vi "Robot Main.vi"() -> ()   [LabVIEW 2018]
doc: "Robot Main serves as the primary scheduler for your command and control robotics program. It should not be necessary to modify this VI. Instead, you should add your code to the VIs called from Robot Main - Teleop, Autonomous, and SubSystems."
uses:
  <vilib>/Rock Robotics/WPI/Camera/WPI_CameraImageSize.ctl
  Drive/Implementation/Drive Operations.ctl
  <vilib>/Rock Robotics/SystemInterfaces/NetworkCommunication/NetComm_UsageReport_ResourceType.ctl
  Framework/Robot Global Data.vi
  LattePanda/Implementation/LattePanda Published Globals.vi
  <vilib>/Rock Robotics/Network Tables/NT Write Number.vi
  <vilib>/Rock Robotics/Network Tables/NT Read String.vi
  <vilib>/Rock Robotics/Network Tables/NT Write Variant.vi
panel:
  out "Path Data":refnum<vi>[](array[refnum])
  out "LattePanda Connected":bool
  in  "Operation":T1=enum."Immediate"
  in  "Image Size":T2=enum."320x240"
  in  "Finish":bool
  # "1. Get the camera mounted on the back\n2. Clean up Elevator Teleop"
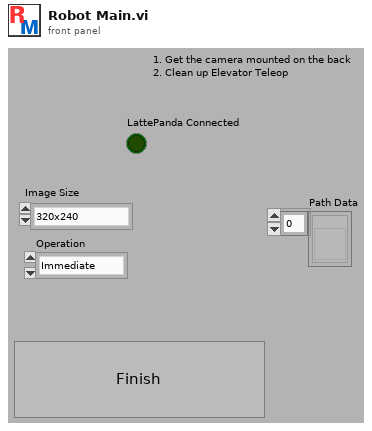
[diagram p1: front panel]
types:
  T1 = typedef "Drive Operations.ctl" = enum16{"Reserve", "Read Current", "Immediate", "J-Turn", "Play Back From Log", "Auto-Align"}
  T2 = typedef "WPI_CameraImageSize.ctl" = enum16{"640x480", "320x240", "160x120", "Custom"}
  T3 = typedef "NetComm_UsageReport_ResourceType.ctl" = enum8{"Controller", "Module", "Language", "CANPlugin", "Accelerometer", "ADXL345", "AnalogChannel", "AnalogTrigger", "AnalogTriggerOutput", "CANJaguar", "Compressor", "Counter", "Dashboard", "DigitalInput", "DigitalOutput", "DriverStationCIO", "DriverStationEIO", "DriverStationLCD", "Encoder", "GearTooth", "Gyro", "I2C", "Framework", "Jaguar", "Joystick", "Kinect", "KinectStick", "PIDController", "Preferences", "PWM", "Relay", "RobotDrive", "SerialPort", "Servo", "Solenoid", "SPI", "Task", "Ultrasonic", "Victor", "Button", "Command", "AxisCamera", "PCVideoServer", "SmartDashboard", "Talon", "HiTechnicColorSensor", "HiTechnicAccel", "HiTechnicCompass", "SRF08", "AnalogOutput", "Victor SP", "Talon SRX", "CAN Talon SRX", "ADXL362 Accel", "ADXRS450 Gyro", "Rev SPARK", "Mindsensors SD540", "Digital Filter", "ADIS16448", "PDP", "PCM", "PigeonIMU", "Nidec Brushless", "CTRE CANifier", "CTRE Future 0", "CTRE Future 1", "CTRE Future 2", "CTRE Future 3", "CTRE Future 4", "CTRE Future 5", "CTRE Future 6", "Linear Filter", "Xbox Controller", "USB Camera", "NavX", "Pixy", "Pixy2", "ScanseSweep", "Shuffleboard", "CAN", "Digilent DMC60", "PWM Victor SPX", "Rev SPARK MAX PWM", "Rev SPARK MAX CAN", "ADIS16470"}
  T4 = cluster{"Segment Name":string, "Type":enum16{"Accel Straight", "Const Straight", "Blend", "Circle"}, "Traj Pos Points":cluster{"x":dbl, "y":dbl, "th":dbl}[], "Traj Vel Points":cluster{"V":dbl, "th":dbl}[], "Accel Index":i32, "Decel Index":i32}[]
  T5 = cluster{"Points":cluster{"x":dbl, "y":dbl, "th":dbl}[], "Trajectory Data":cluster{"Segment Name":string, "Type":enum16{"Accel Straight", "Const Straight", "Blend", "Circle"}, "Traj Pos Points":cluster{"x":dbl, "y":dbl, "th":dbl}[], "Traj Vel Points":cluster{"V":dbl, "th":dbl}[], "Accel Index":i32, "Decel Index":i32}[]}
  T6 = typedef "ADIS16448_IMU.lvlib/ADI_IMU_ADIS16448_IMUDevRef.ctl" = cluster{"DevStatus":errorcluster, "Handle":i32, "SPI Bus":T7, "Device Found":bool, "Device Ready":bool, "Yaw Axis":enum16{"X", "Y", "Z"}, "AHRS Algorithm":enum16{"Complementary", "Madgwick"}, "Serial":u16, "Lot ID 2":u16, "Lot ID 1":u16, "Bytes Per Sample":u16, "Calibrate On Open?":bool}
  T7 = typedef "spi_bus.ctl" = enum16{"SPI On-Board, CS0", "SPI On-Board, CS1", "SPI On-Board, CS2", "SPI On-Board, CS3", "SPI MXP", "Invalid"}
  T8 = typedef "WPI_JoystickDevRef.ctl" = cluster{"Device":T9}
  T9 = typedef "WPI_JoystickDeviceEnum.ctl" = enum16{"USB 0", "USB 1", "USB 2", "USB 3", "USB 4", "USB 5"}
  T10 = typedef "WPI_DriverStationMatch Info.ctl" = cluster{"Autonomous Elapsed Seconds":dbl, "TeleOp Elapsed Seconds":dbl, "Disabled Elapsed Seconds":dbl, "Visited Autonomous":bool, "Visited TeleOp":bool, "Visited Disabled":bool, "Autonomous Settings":cluster{"Autonomous Style":enum16{"Iterative", "Independent"}, "VI Refnum":refnum<vi>}}
  T11 = typedef "WPI_DriverStationDerivedRobotMode.ctl" = enum16{"Init", "Execute", "Stop"}
  T12 = typedef "WPI_DriverStationRobotMode2.ctl" = enum16{"Autonomous Disabled", "Autonomous Enabled", "Teleop Disabled", "Teleop Enabled", "Disconnected", "Finish", "Test Disabled", "Test Enabled", "Emergency Stopped"}
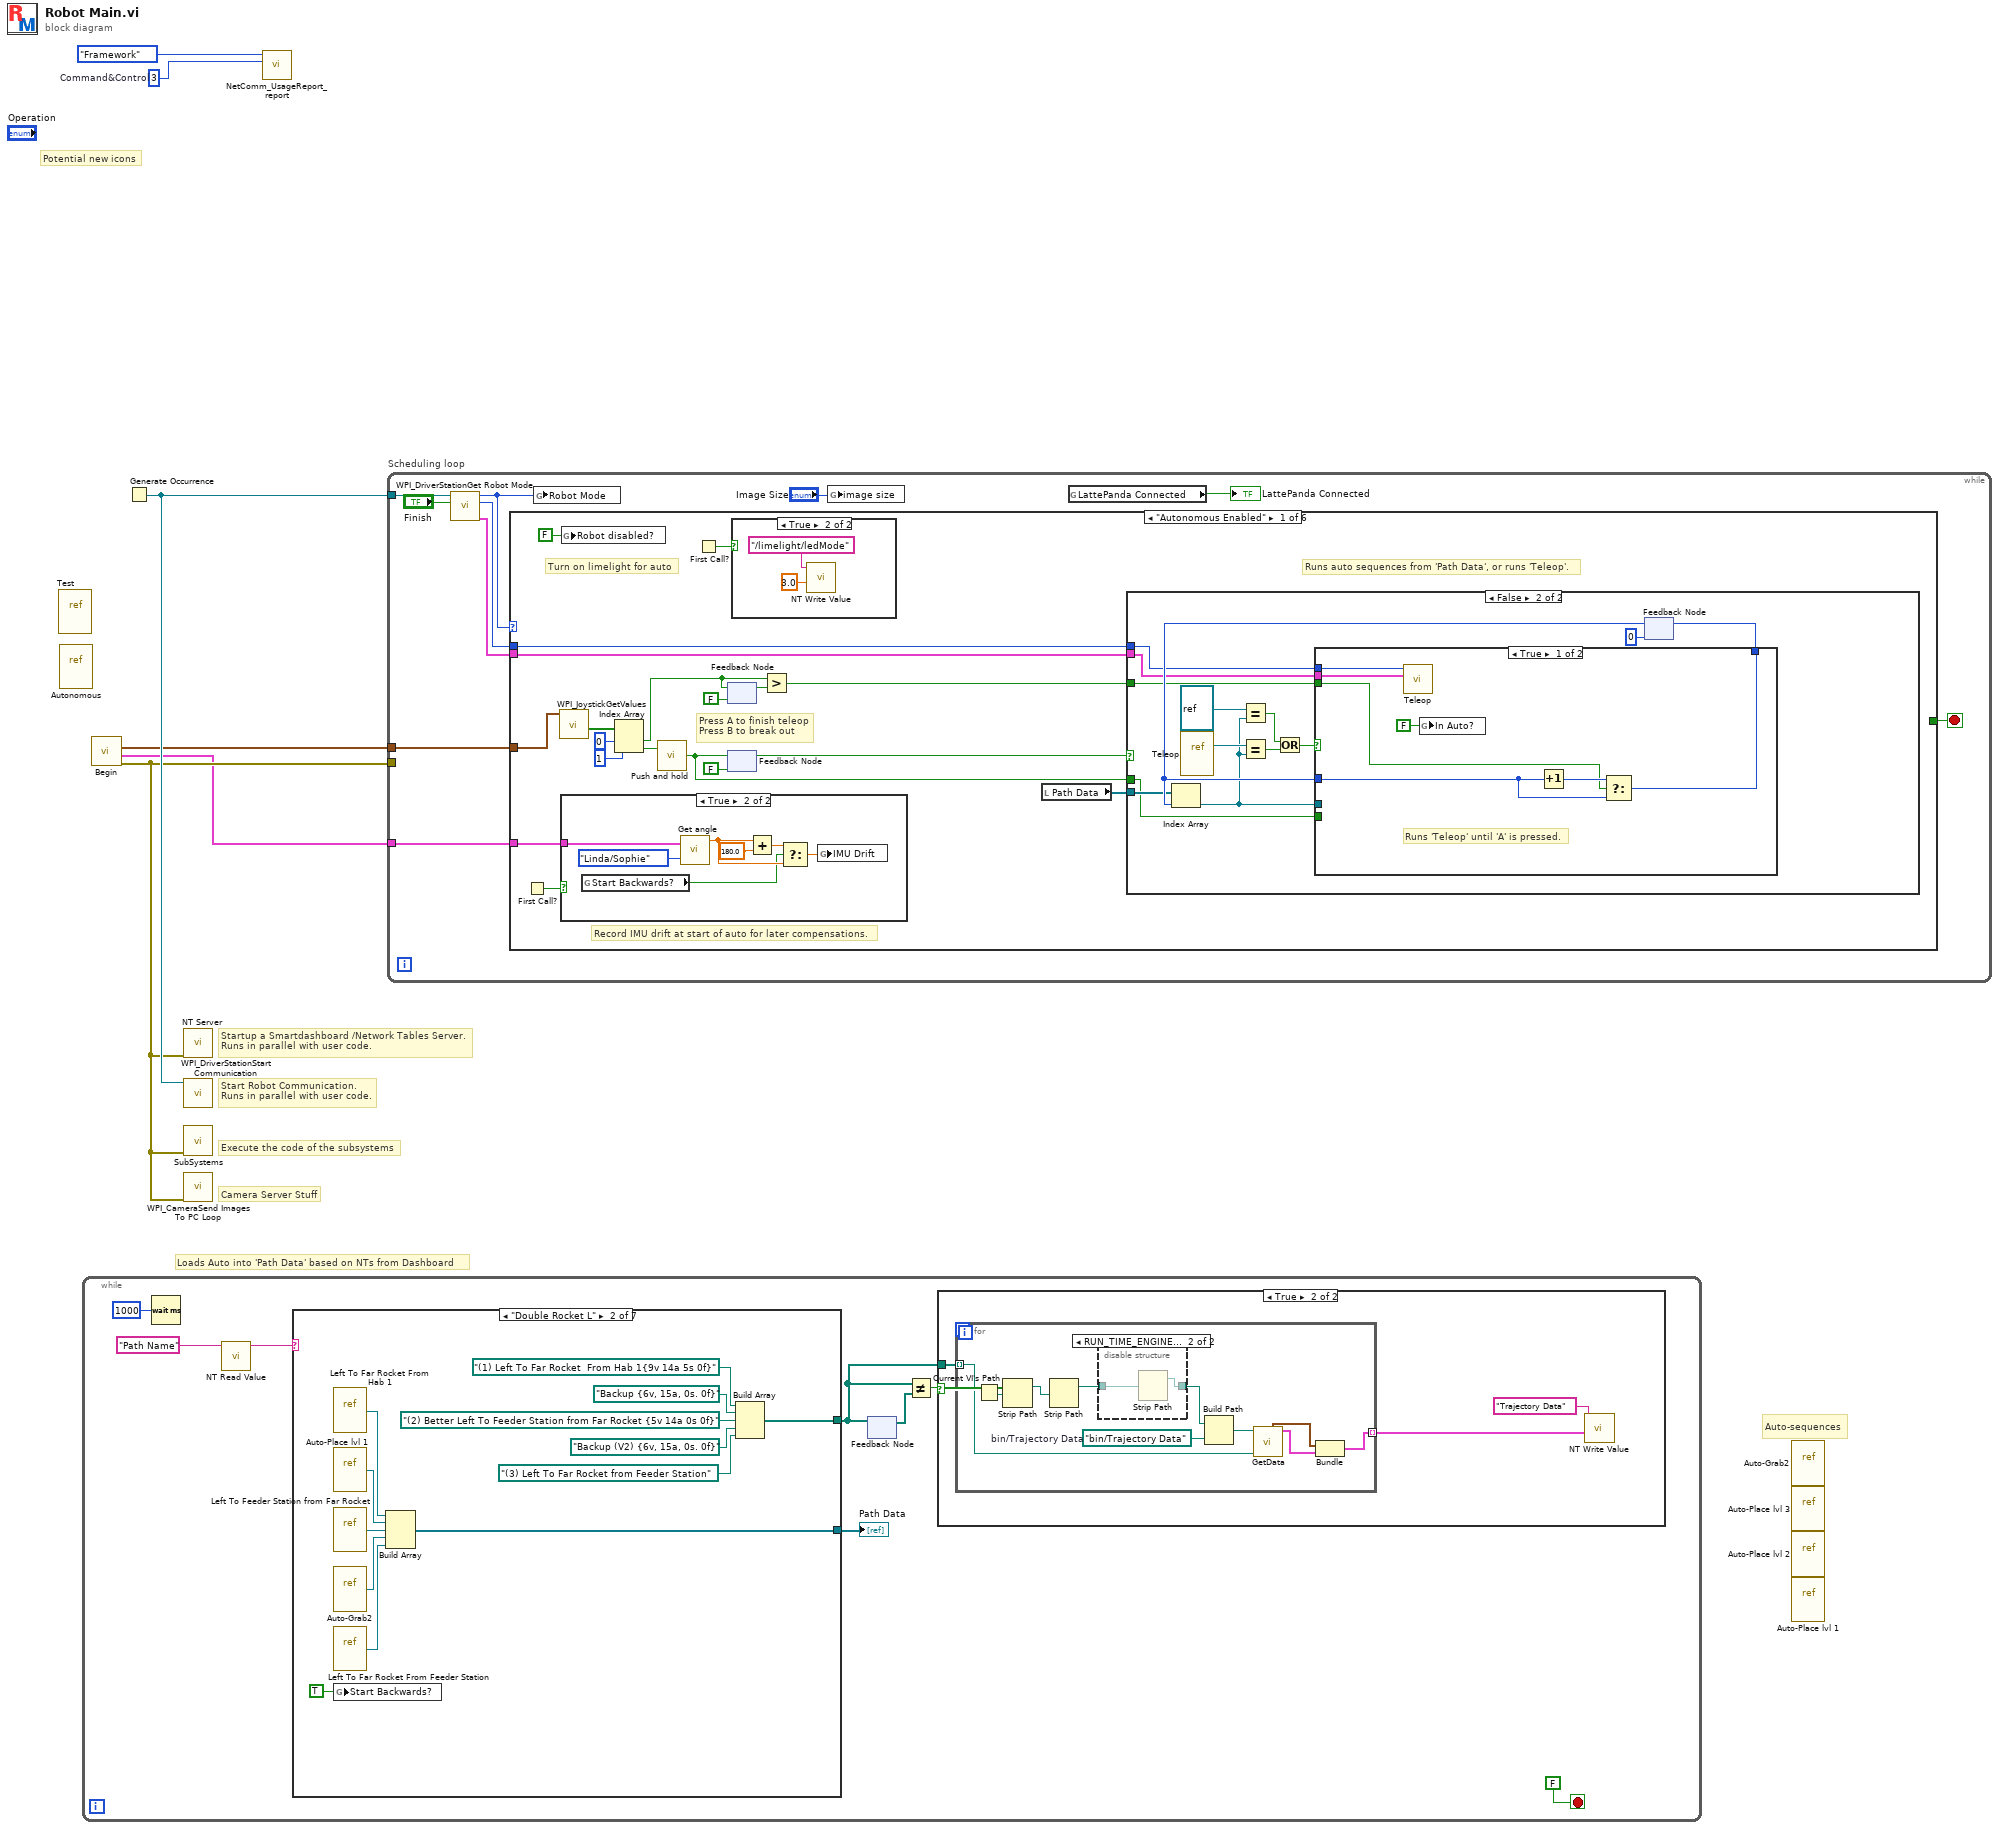
[diagram p0: block diagram]
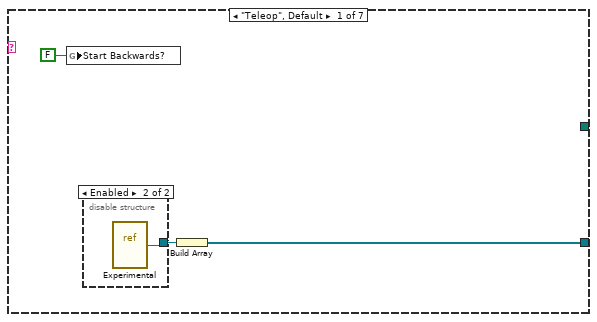
[diagram p4: hidden frame]
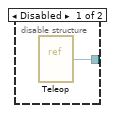
[diagram p5: hidden frame]
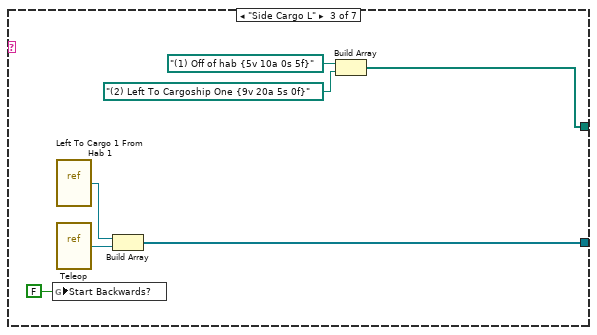
[diagram p6: hidden frame]
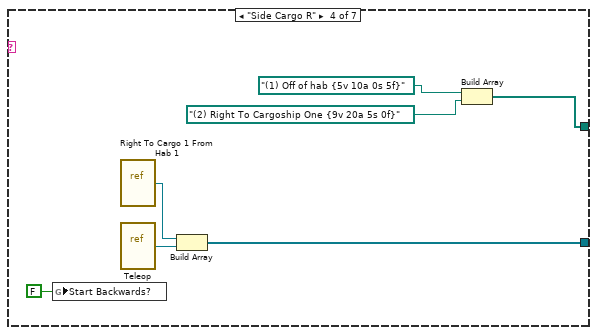
[diagram p7: hidden frame]
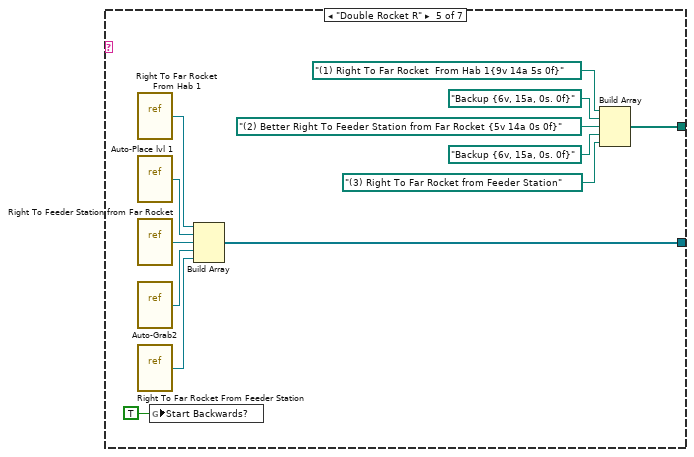
[diagram p8: hidden frame]
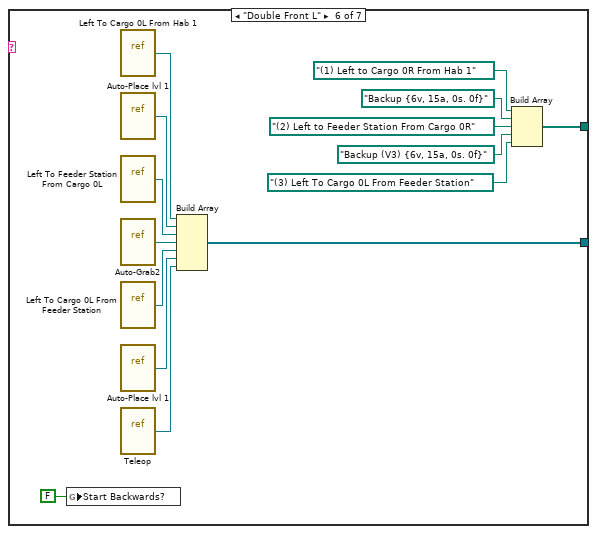
[diagram p9: hidden frame]
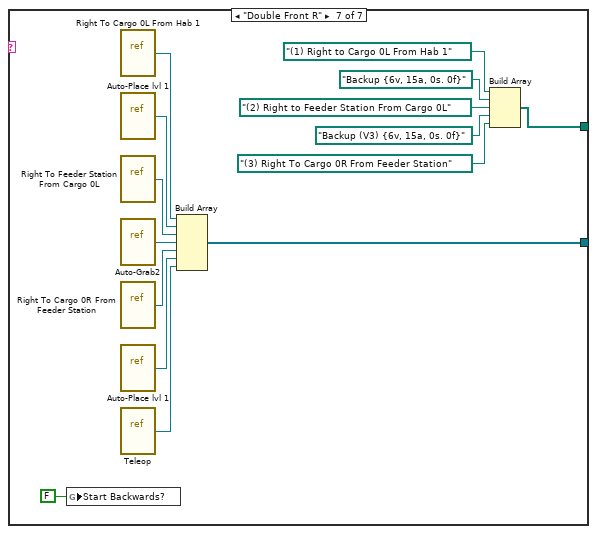
[diagram p10: hidden frame]
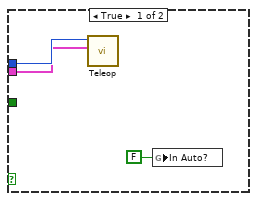
[diagram p13: hidden frame]
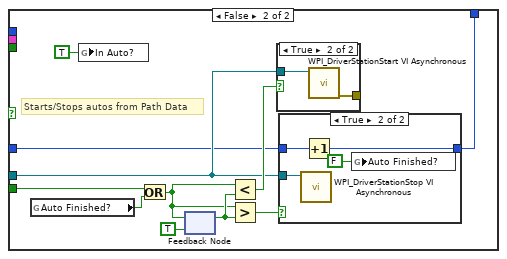
[diagram p14: hidden frame]
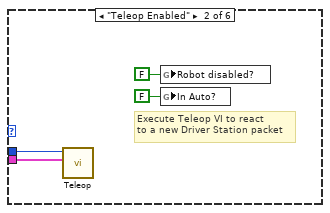
[diagram p17: hidden frame]
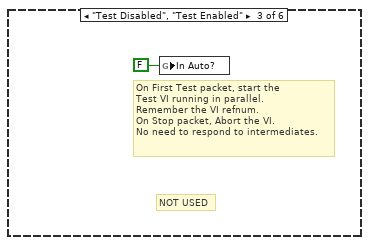
[diagram p18: hidden frame]
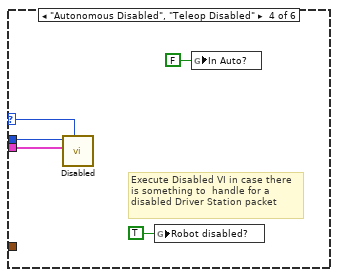
[diagram p19: hidden frame]
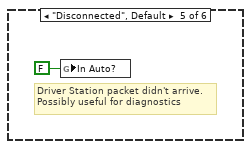
[diagram p20: hidden frame]
diagram:
  w4 = u8 3  # Command&Control
  # "Loads Auto into 'Path Data' based on NTs from Dashboard"
  # "Camera Server Stuff"
  # "Auto-sequences"
  # "Startup a Smartdashboard /Network Tables Server.\nRuns in parallel with user code."
  # "Potential new icons"
  # "Execute the code of the subsystems"
  # "Start Robot Communication.\nRuns in parallel with user code."
  n1 = vi-ref "Test.vi"() -> ()  [unwired: 1 out]
  n2 = vi-ref "Autonomous.vi"() -> ()  [unwired: 1 out]
  n3 = while {
    stop <- FALSE stop-if-true
    n4 = Wait (ms)(milliseconds to wait=u32 1000) -> ()  [unwired: 1 out]
    n5 = call-poly <vilib>:"NT Read Value.vi"("Name"="Path Name") -> ("String"=w13:string)  [unwired: 9 in, 1 out]
    n6 = case shown="\"Double Rocket L\"" w13 {
      tunnel: [w32 w48 w55 w62 w75 w90 w105] -> w10
      tunnel: [_ w36 w50 w56 w63 w76 w91] -> w7
      frame "Teleop", Default {
        n7 = global write "Robot Global Data.vi" "Start Backwards?"(FALSE ("Start Backwards?")) -> ()
        n8 = disable-structure shown="Enabled" {
          disable-tunnel: [w34 w35] -> w33
          frame Disabled {
            n9 = vi-ref "Teleop.vi"() -> (w34:refnum<vi>)
          }
          frame Enabled {
            n10 = vi-ref "Experimental.vi"() -> (w35:refnum<vi>)
          }
        }
        n11 = Build Array(w33) -> (w32:refnum<vi>[])
      }
      frame "Double Rocket L" {
        n12 = vi-ref "Left To Far Rocket From Hab 1.vi"() -> (w46:refnum<vi>)
        n13 = vi-ref "Auto-Place lvl 1.vi"() -> (w42:refnum<vi>)
        n14 = vi-ref "Left To Feeder Station from Far Rocket.vi"() -> (w45:refnum<vi>)
        n15 = vi-ref "Auto-Grab2.vi"() -> (w44:refnum<vi>)
        n16 = vi-ref "Left To Far Rocket From Feeder Station.vi"() -> (w47:refnum<vi>)
        n17 = global write "Robot Global Data.vi" "Start Backwards?"(TRUE ("Start Backwards?")) -> ()
        n18 = Build Array(w46, w42, w45, w44, w47) -> (w48:refnum<vi>[])
        n19 = Build Array(path "(1) Left To Far Rocket  From Hab 1{9v 14a 5s 0f}", path "Backup {6v, 15a, 0s. 0f}", path "(2) Better Left To Feeder Station from Far Rocket {5v 14a 0s 0f}", path "Backup (V2) {6v, 15a, 0s. 0f}", path "(3) Left To Far Rocket from Feeder Station") -> (w36:path[])
      }
      frame "Side Cargo L" {
        n20 = global write "Robot Global Data.vi" "Start Backwards?"(FALSE ("Start Backwards?")) -> ()
        n21 = vi-ref "Left To Cargo 1 From Hab 1.vi"() -> (w53:refnum<vi>)
        n22 = vi-ref "Teleop.vi"() -> (w52:refnum<vi>)
        n23 = Build Array(w53, w52) -> (w55:refnum<vi>[])
        n24 = Build Array(path "(1) Off of hab {5v 10a 0s 5f}", path "(2) Left To Cargoship One {9v 20a 5s 0f}") -> (w50:path[])
      }
      frame "Side Cargo R" {
        n25 = global write "Robot Global Data.vi" "Start Backwards?"(FALSE ("Start Backwards?")) -> ()
        n26 = vi-ref "Right To Cargo 1 From Hab 1.vi"() -> (w59:refnum<vi>)
        n27 = vi-ref "Teleop.vi"() -> (w60:refnum<vi>)
        n28 = Build Array(w59, w60) -> (w62:refnum<vi>[])
        n29 = Build Array(path "(1) Off of hab {5v 10a 0s 5f}", path "(2) Right To Cargoship One {9v 20a 5s 0f}") -> (w56:path[])
      }
      frame "Double Rocket R" {
        n30 = vi-ref "Right To Far Rocket From Hab 1.vi"() -> (w73:refnum<vi>)
        n31 = vi-ref "Auto-Place lvl 1.vi"() -> (w69:refnum<vi>)
        n32 = vi-ref "Right To Feeder Station from Far Rocket.vi"() -> (w72:refnum<vi>)
        n33 = vi-ref "Auto-Grab2.vi"() -> (w70:refnum<vi>)
        n34 = vi-ref "Right To Far Rocket From Feeder Station.vi"() -> (w74:refnum<vi>)
        n35 = global write "Robot Global Data.vi" "Start Backwards?"(TRUE ("Start Backwards?")) -> ()
        n36 = Build Array(w73, w69, w72, w70, w74) -> (w75:refnum<vi>[])
        n37 = Build Array(path "(1) Right To Far Rocket  From Hab 1{9v 14a 5s 0f}", path "Backup {6v, 15a, 0s. 0f}", path "(2) Better Right To Feeder Station from Far Rocket {5v 14a 0s 0f}", path "Backup {6v, 15a, 0s. 0f}", path "(3) Right To Far Rocket from Feeder Station") -> (w63:path[])
      }
      frame "Double Front L" {
        n38 = global write "Robot Global Data.vi" "Start Backwards?"(FALSE ("Start Backwards?")) -> ()
        n39 = vi-ref "Left To Cargo 0L From Hab 1.vi"() -> (w88:refnum<vi>)
        n40 = vi-ref "Auto-Place lvl 1.vi"() -> (w87:refnum<vi>)
        n41 = vi-ref "Left To Feeder Station From Cargo 0L.vi"() -> (w86:refnum<vi>)
        n42 = vi-ref "Auto-Grab2.vi"() -> (w85:refnum<vi>)
        n43 = vi-ref "Left To Cargo 0L From Feeder Station.vi"() -> (w84:refnum<vi>)
        n44 = vi-ref "Auto-Place lvl 1.vi"() -> (w83:refnum<vi>)
        n45 = vi-ref "Teleop.vi"() -> (w82:refnum<vi>)
        n46 = Build Array(w88, w87, w86, w85, w84, w83, w82) -> (w90:refnum<vi>[])
        n47 = Build Array(path "(1) Left to Cargo 0R From Hab 1" ("Path"), path "Backup {6v, 15a, 0s. 0f}", path "(2) Left to Feeder Station From Cargo 0R", path "Backup (V3) {6v, 15a, 0s. 0f}", path "(3) Left To Cargo 0L From Feeder Station") -> (w76:path[])
      }
      frame "Double Front R" {
        n48 = global write "Robot Global Data.vi" "Start Backwards?"(FALSE ("Start Backwards?")) -> ()
        n49 = vi-ref "Right To Cargo 0L From Hab 1.vi"() -> (w103:refnum<vi>)
        n50 = vi-ref "Auto-Place lvl 1.vi"() -> (w102:refnum<vi>)
        n51 = vi-ref "Right To Feeder Station From Cargo 0L.vi"() -> (w101:refnum<vi>)
        n52 = vi-ref "Auto-Grab2.vi"() -> (w100:refnum<vi>)
        n53 = vi-ref "Right To Cargo 0R From Feeder Station.vi"() -> (w99:refnum<vi>)
        n54 = vi-ref "Auto-Place lvl 1.vi"() -> (w98:refnum<vi>)
        n55 = vi-ref "Teleop.vi"() -> (w97:refnum<vi>)
        n56 = Build Array(w103, w102, w101, w100, w99, w98, w97) -> (w105:refnum<vi>[])
        n57 = Build Array(path "(1) Right to Cargo 0L From Hab 1" ("Path"), path "Backup {6v, 15a, 0s. 0f}", path "(2) Right to Feeder Station From Cargo 0L", path "Backup (V3) {6v, 15a, 0s. 0f}", path "(3) Right To Cargo 0R From Feeder Station") -> (w91:path[])
      }
    }
    "Path Data" <- w10
    n58 = feedback-in #1(w7) -> ()
    n59 = feedback #1() -> (w9:path[])  [unwired: 1 in]
    n60 = Not Equal?(x=w7, y=w9) -> (x != y?=w8:bool)
    n61 = case shown="True" w8 {
      tunnel: w7 -> [_ w17]
      frame False {
      }
      frame True {
        n62 = for {
          tunnel: w17 -> [w20] mode=indexing
          tunnel: [w22] -> w15 mode=indexing
          w21 = path "bin/Trajectory Data"  # bin/Trajectory Data
          n63 = Current VI's Path() -> (path=w19:path)
          n64 = Strip Path(path=w19) -> (stripped path=w26:path)  [unwired: 1 out]
          n65 = Strip Path(path=w26) -> (stripped path=w25:path)  [unwired: 1 out]
          n66 = disable-structure shown="RUN_TIME_ENGINE==True, Default" {
            disable-tunnel: [w28 w29] -> w18
            disable-tunnel: w25 -> [w28 w30]
            frame condition #0 (active) {
            }
            frame condition #1 {
              n67 = Strip Path(path=w30) -> (stripped path=w29:path)  [unwired: 1 out]
            }
          }
          n68 = Build Path(base path=w18, name or relative path=w21) -> (appended path=w27:path)
          n69 = call "GetData.vi"("File"=w20, "file (use dialog)"=w27) -> ("Trajectory Data"=w23:T4, "Points"=w24:cluster{"x":dbl, "y":dbl, "th":dbl}[])  [unwired: 2 in, 6 out]
          n70 = Bundle("Points"=w24, "Trajectory Data"=w23) -> (w22:T5)  [unwired: 1 in]
        }
        n71 = call-poly <vilib>:"NT Write Value.vi"("Variant"=w15, "Name"="Trajectory Data") -> ()  [unwired: 9 in, 1 out]
      }
    }
  }
  n72 = call "Begin.vi"() -> ("error out"=w3:errorcluster, "ADI IMU DevRef"=w1:T6, "JoystickDevRef"=w2:T8)  [unwired: 2 in, 7 out]
  n73 = Generate Occurrence() -> (w6:refnum<k4>)
  n74 = call <vilib>:"NT Server.vi"("error in (no error)"=w3) -> ()  [unwired: 11 in]
  n75 = call <vilib>:"WPI_DriverStationStart Communication.vi"("occurrence"=w6) -> ()  [unwired: 1 in, 10 out]
  n76 = call "SubSystems.vi"("error in"=w3) -> ()  [unwired: 11 in]
  n77 = call <vilib>:"WPI_CameraSend Images To PC Loop.vi"("error in (no error)"=w3) -> ()  [unwired: 11 in]
  n78 = call <vilib>:"NetComm_UsageReport_report.vi"("Instance Number"=w4, "Resource Type"=NetComm_UsageReport_ResourceType."Framework") -> ()  [unwired: 10 in]
  n79 = while "Scheduling loop" {
    tunnel: w6 -> [w114]
    tunnel: w3 -> [_]
    tunnel: w2 -> [w107]
    tunnel: w1 -> [w106]
    stop <- w111 stop-if-true
    n80 = call <vilib>:"WPI_DriverStationGet Robot Mode.vi"("Finish"="Finish", "DS Occurrence"=w114) -> ("Match Info out"=w112:T10, "Call Context"=w115:T11, "Robot Mode"=w110:T12)  [unwired: 7 out]
    n81 = case shown="\"Autonomous Enabled\"" w110 {
      selector: w110 -> [_ _ _ w193 _ _]
      tunnel: w115 -> [w133 w189 _ w195 _ _]
      tunnel: w112 -> [w132 w188 _ w194 _ _]
      tunnel: [_ _ _ _ _ TRUE] -> w111
      tunnel: w107 -> [w134 _ _ _ _ _]
      tunnel: w106 -> [w131 _ _ _ _ _]
      frame "Autonomous Enabled" {
        # "Runs auto sequences from 'Path Data', or runs 'Teleop'."
        # "Record IMU drift at start of auto for later compensations."
        # "Turn on limelight for auto"
        # "Press A to finish teleop\nPress B to break out"
        n82 = First Call?() -> (First Call?: T/F=w129:bool)
        n83 = call <vilib>:"WPI_JoystickGetValues.vi"("JoystickDevRef"=w134) -> ("Buttons"=w128:bool[])  [unwired: 6 in, 4 out]
        n84 = case shown="True" w129 {
          tunnel: w131 -> [_ w142]
          frame False {
          }
          frame True {
            n85 = global read "Robot Global Data.vi" "Start Backwards?"() -> (w137:bool)
            n86 = call "Get angle.vi"("ADI IMU DevRef Out"=w142, "Robot"=enum16{"Linda/Sophie", "Mule"}."Linda/Sophie") -> ("Out"=w138:dbl)  [unwired: 2 out]
            n87 = Add(x=w138, y=180.0) -> (x+y=w140:dbl)
            n88 = Select(t=w140, s=w137, f=w138) -> (s? t:f=w139:dbl)
            n89 = global write "Robot Global Data.vi" "IMU Drift"(w139) -> ()
          }
        }
        n90 = global write "Robot Global Data.vi" "Robot disabled?"(FALSE ("Robot disabled?")) -> ()
        n91 = Index Array(array=w128, index #1=0 ("index"), index #2=1 ("index")) -> (element #1=w120:bool, element #2=w122:bool)
        n92 = call "Push and hold.vi"("Input"=w122) -> ("Output"=w125:bool)  [unwired: 1 in]
        n93 = First Call?() -> (First Call?: T/F=w117:bool)
        n94 = feedback-in #2(w120) -> ()
        n95 = feedback #2(FALSE) -> (w121:bool)
        n96 = feedback #3(FALSE ("Output")) -> (w126:bool)
        n97 = feedback-in #3(w125) -> ()
        n98 = case shown="True" w117 {
          frame False {
          }
          frame True {
            n99 = call-poly <vilib>:"NT Write Value.vi"("Numeric"=3.0, "Name"="/limelight/ledMode") -> ()  [unwired: 9 in, 1 out]
          }
        }
        n100 = Greater?(x=w120, y=w121) -> (0:w119:bool)
        n101 = local read "Path Data"() -> (w116:refnum<vi>[])
        n102 = case shown="False" w126 {
          tunnel: w116 -> [_ w157]
          tunnel: w125 -> [_ w156]
          tunnel: w133 -> [w145 w154]
          tunnel: w132 -> [w144 w153]
          tunnel: w119 -> [_ w152]
          frame True {
            n103 = call "Teleop.vi"("Match Info"=w144, "Call Context"=w145) -> ()  [unwired: 1 in, 9 out]
            n104 = global write "Robot Global Data.vi" "In Auto?"(FALSE ("In Auto?")) -> ()
          }
          frame False {
            n105 = vi-ref "Teleop.vi"() -> (w155:refnum<vi>)
            n106 = feedback #4(0) -> (w159:i32)
            n107 = Index Array(array=w157, index=w159) -> (element=w148:refnum<vi>)
            n108 = Equal?(x=refnum<vi> refnum, y=w148) -> (x = y?=w151:bool)
            n109 = Equal?(x=w155, y=w148) -> (x = y?=w150:bool)
            n110 = Or(x=w151, y=w150) -> (x .or. y?=w147:bool)
            n111 = case shown="True" w147 {
              tunnel: w148 -> [_ w175]
              tunnel: [w163 w174] -> w160
              tunnel: w159 -> [w162 w173]
              tunnel: w156 -> [_ w169]
              tunnel: w154 -> [w167 _]
              tunnel: w153 -> [w166 _]
              tunnel: w152 -> [w161 _]
              frame True {
                # "Runs 'Teleop' until 'A' is pressed."
                n112 = call "Teleop.vi"("Match Info"=w166, "Call Context"=w167) -> ()  [unwired: 1 in, 9 out]
                n113 = global write "Robot Global Data.vi" "In Auto?"(FALSE ("In Auto?")) -> ()
                n114 = Increment(x=w162) -> (x+1=w164:i32)
                n115 = Select(t=w164, s=w161, f=w162) -> (s? t:f=w163:i32)
              }
              frame False {
                # "Starts/Stops autos from Path Data"
                n116 = global read "Robot Global Data.vi" "Auto Finished?"() -> (w171:bool)
                n117 = global write "Robot Global Data.vi" "In Auto?"(TRUE ("In Auto?")) -> ()
                n118 = Or(x=w169, y=w171) -> (x .or. y?=w170:bool)
                n119 = feedback #5(TRUE ("Auto Finished?")) -> (w177:bool)
                n120 = feedback-in #5(w170) -> ()
                n121 = Less?(x=w170, y=w177) -> (x < y?=w176:bool)
                n122 = Greater?(x=w170, y=w177) -> (0:w178:bool)
                n123 = case shown="True" w176 {
                  tunnel: w175 -> [_ w180]
                  tunnel: [_ w179] -> _
                  frame False {
                  }
                  frame True {
                    n124 = call <vilib>:"WPI_DriverStationStart VI Asynchronous.vi"("VI"=w180) -> ("error out"=w179:errorcluster)  [unwired: 10 out]
                  }
                }
                n125 = case shown="True" w178 {
                  tunnel: w175 -> [_ w185]
                  tunnel: [w181 w183] -> w174
                  tunnel: w173 -> [w181 w184]
                  frame False {
                  }
                  frame True {
                    n126 = call <vilib>:"WPI_DriverStationStop VI Asynchronous.vi"("VI Refnum"=w185) -> ()  [unwired: 11 out]
                    n127 = Increment(x=w184) -> (x+1=w183:i32)
                    n128 = global write "Robot Global Data.vi" "Auto Finished?"(FALSE ("Auto Finished?")) -> ()
                  }
                }
              }
            }
            n129 = feedback-in #4(w160) -> ()
          }
        }
      }
      frame "Teleop Enabled" {
        # "Execute Teleop VI to react\nto a new Driver Station packet"
        n130 = call "Teleop.vi"("Match Info"=w188, "Call Context"=w189) -> ()  [unwired: 1 in, 9 out]
        n131 = global write "Robot Global Data.vi" "Robot disabled?"(FALSE ("Robot disabled?")) -> ()
        n132 = global write "Robot Global Data.vi" "In Auto?"(FALSE ("In Auto?")) -> ()
      }
      frame "Test Disabled", "Test Enabled" {
        # "NOT USED"
        # "On First Test packet, start the\nTest VI running in parallel.\nRemember the VI refnum.\nOn Stop packet, Abort the VI.\nNo need to respond to intermediates."
        n133 = global write "Robot Global Data.vi" "In Auto?"(FALSE ("In Auto?")) -> ()
      }
      frame "Autonomous Disabled", "Teleop Disabled" {
        # "Execute Disabled VI in case there\nis something to  handle for a\ndisabled Driver Station packet"
        n134 = call "Disabled.vi"("Robot Mode"=w193, "Match Info"=w194, "Call Context"=w195) -> ()  [unwired: 1 in, 8 out]
        n135 = global write "Robot Global Data.vi" "Robot disabled?"(TRUE ("Robot disabled?")) -> ()
        n136 = global write "Robot Global Data.vi" "In Auto?"(FALSE ("In Auto?")) -> ()
      }
      frame "Disconnected", Default {
        # "Driver Station packet didn't arrive.\nPossibly useful for diagnostics"
        n137 = global write "Robot Global Data.vi" "In Auto?"(FALSE ("In Auto?")) -> ()
      }
      frame "Finish" {
        # "Call  Finish VI and\nexit the loop"
        n138 = global write "Robot Global Data.vi" "In Auto?"(FALSE ("In Auto?")) -> ()
        n139 = call "Finish.vi"() -> ()  [unwired: 1 in, 7 out]
      }
    }
    n140 = global write "Robot Global Data.vi" "Robot Mode"(w110) -> ()
    n141 = global write "Robot Global Data.vi" "image size"("Image Size") -> ()
    n142 = global read "LattePanda Published Globals.vi" "LattePanda Connected"() -> (→"LattePanda Connected":bool)
  }
  n143 = vi-ref "Auto-Grab2.vi"() -> ()  [unwired: 1 out]
  n144 = vi-ref "Auto-Place lvl 3.vi"() -> ()  [unwired: 1 out]
  n145 = vi-ref "Auto-Place lvl 2.vi"() -> ()  [unwired: 1 out]
  n146 = vi-ref "Auto-Place lvl 1.vi"() -> ()  [unwired: 1 out]
